vi "YOLOv8_OBB_OpenVINO_NIVision_img.vi"() -> ()   [LabVIEW 2018]
doc: "YOLOv8_OBB_OpenVINO_NIVision_img: This example demonstrates the integration of YOLOv8 with OpenVINO and the NI Vision library for object detection with oriented bounding boxes (OBB) in images. The YOLOv8 model detects objects in images and outputs precise oriented bounding boxes, which indicate both the position and orientation of the detected objects. The NI Vision library is used for advanced image processing tasks such as capturing, filtering, and analyzing the input image, while OpenVINO ensures fast, optimized inference on Intel hardware. This solution is ideal for applications where accurate localization of rotated or irregularly shaped objects is required, such as in industrial automation, robotics, or quality control, with real-time performance and scalability across multiple platforms."
uses:
  vi.lib/VIRobotics/ModelZoo/Object_Detection/yolov8_obb_openvino/Initial_yolov8_Obb_OpenVINO.vi
  vi.lib/VIRobotics/ModelZoo/Object_Detection/yolov8_obb_openvino/yolov8_obb_openvino.lvclass
panel:
  in  "pic_path":path=path "C:/ProgramData/VIRobotics/ModelZoo/Object_Detection/imgs/test.png"
  in  "device_name":string(combo)="CPU"
  in  "class_names_file":path=path "C:/ProgramData/VIRobotics/ModelZoo/Object_Detection/coco.names"
  in  "model_file":path=path "C:/ProgramData/VIRobotics/ModelZoo/Object_Detection/yolov8_obb/onnx_model/yolov8n-obb.onnx"
  out "Image":T1(plugin-control)
  out "每帧耗时(s)":dbl
  # "Overview: Demonstrates how to use the VIRobotics OpenVINO toolkit to load the the ONNX model of yolov8_obb for  object detection.\nRequirements: Windows.\nInstructions: \n1.Select the device_name to use.（If your computer has Intel GPU, you can select GPU in the \"type\" control before running the VI to achieve faster inference).\n2.Specify the pic_path\n3.Run the VI.\nIf you want to load the model you trained, follow the following steps:\n1.Select the device_name to use. \n2.Specify the model_file and class_names_file.\n3.Specify the pic_path\n4.Run the VI."
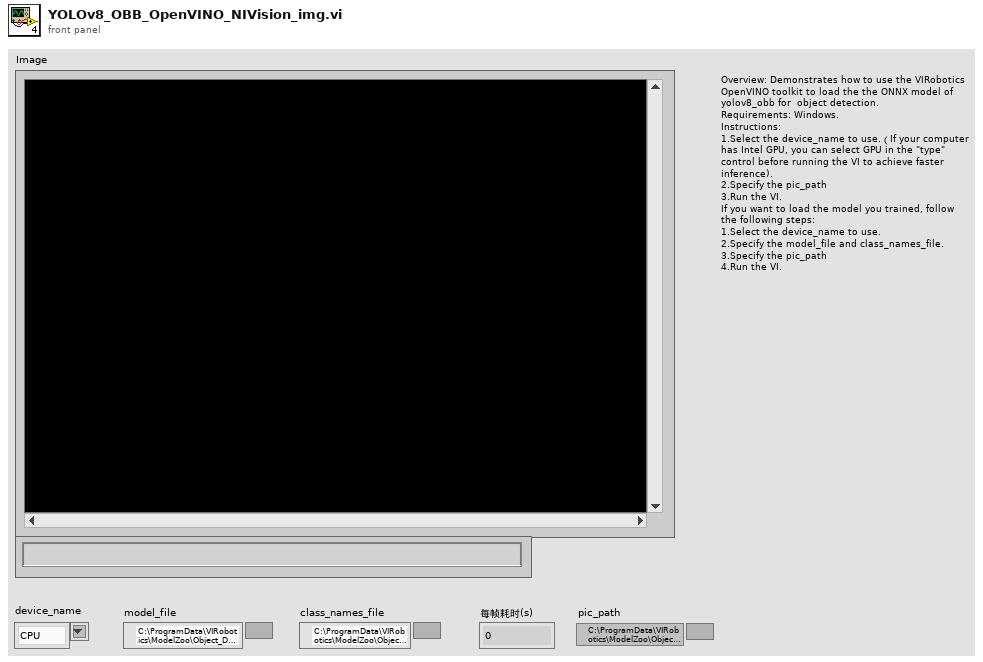
[diagram p1: front panel]
types:
  T1 = typedef "IMAQ Image.ctl" = refnum<image>
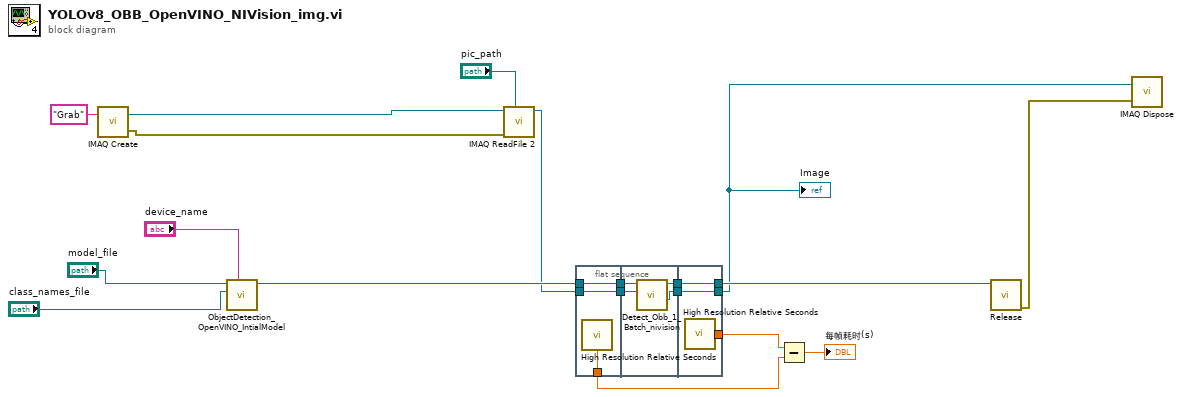
[diagram p0: block diagram]
diagram:
  n1 = call "IMAQ Create"("Image Name"="Grab") -> ("New Image"=w6:T1, "error out"=w5:errorcluster)  [unwired: 3 in, 1 out]
  n2 = call-poly "ObjectDetection_OpenVINO_IntialModel.vi"("device_name"="device_name", "class_names_path"="class_names_file", "path"="model_file") -> ("yolov8_obb_ov out"=w18:refnum<class "yolov8_obb_openvino.lvclass">)  [unwired: 7 in, 1 out]
  n3 = call "IMAQ ReadFile 2"("File Path"="pic_path", "error in (no error)"=w5, "Image"=w6) -> ("Image Out"=w2:T1)  [unwired: 4 in, 4 out]
  n4 = flat-sequence {
    tunnel: w2 -> [w21]
    tunnel: w18 -> [w22]
    tunnel: [w22] -> w14
    tunnel: [w21] -> w13
    tunnel: [w20] -> w10
    tunnel: [w24] -> w12
    tunnel: [w23] -> w11
    tunnel: w14 -> [w26]
    tunnel: w13 -> [w25]
    tunnel: [w28] -> w4
    tunnel: [w29] -> w19
    tunnel: w12 -> [w29]
    tunnel: w11 -> [w28]
    tunnel: [w27] -> w9
    frame #0 {
      n5 = call <vilib>:"High Resolution Relative Seconds.vi"() -> ("relative seconds"=w20:dbl)
    }
    frame #1 {
      n6 = call-dynamic "Detect_Obb_1_Batch_nivision.vi"("Image"=w25, "yolov8_obb_openvino in"=w26) -> ("Image out"=w23:T1, "yolov8_obb_openvino out"=w24:refnum<class "yolov8_obb_openvino.lvclass">)  [unwired: 6 in, 2 out]
    }
    frame #2 {
      n7 = call <vilib>:"High Resolution Relative Seconds.vi"() -> ("relative seconds"=w27:dbl)
    }
  }
  n8 = Subtract(x=w9, y=w10) -> (x-y=→"每帧耗时(s)":dbl)
  n9 = call-dynamic "Release.vi"("yolov8_obb_openvino in"=w19) -> ("error out"=w3:errorcluster)  [unwired: 9 in, 1 out]
  n10 = call "IMAQ Dispose"("Image"=w4, "error in (no error)"=w3) -> ()  [unwired: 4 in, 1 out]
  "Image" <- w4
